vi "配置写入.vi"(8 "error in (no error)":errorcluster caption="错误输入（无错误）") -> (0 "错误输出":errorcluster)   [LabVIEW 2022 SP3, in "斯坦道氨氮V2.lvlib"]
uses:
  <vilib>/Utility/config.llb/NI_LVConfig.lvlib
  <userlib>/_OpenG.lib/variantconfig/variantconfig.llb/openg_variant_configuration_file.lvlib
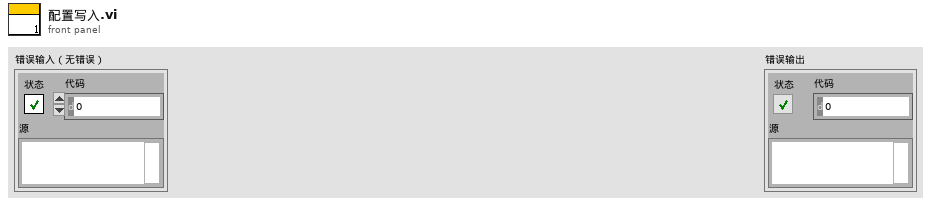
[diagram p1: front panel]
types:
  T1 = typedef "NI_LVConfig.lvlib/Config Data RefNum.ctl" = refnum<k1>
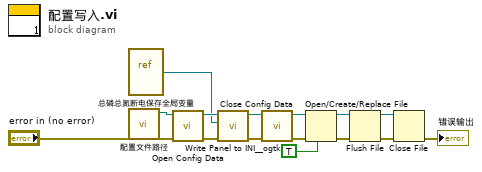
[diagram p0: block diagram]
diagram:
  n1 = vi-ref "总磷总氮断电保存全局变量.vi"() -> (w14:refnum<vi>)
  n2 = call "配置文件路径.vi"() -> ("appended path"=w2:path)  [unwired: 11 in]
  n3 = call <vilib>:"Open Config Data.vi"("error in (no error)"="error in (no error)", "configuration file path"=w2) -> ("error out"=w12:errorcluster, "refnum"=w15:T1)  [unwired: 7 in, 1 out]
  n4 = call <userlib>:"Write Panel to INI__ogtk.vi"("error in (no error)"=w12, "VI ref"=w14, "refnum"=w15) -> ("error out"=w11:errorcluster, "refnum out"=w13:T1)  [unwired: 7 in]
  n5 = call <vilib>:"Close Config Data.vi"("error in (no error)"=w11, "refnum"=w13) -> ("error out"=w6:errorcluster, "file path"=w5:path)  [unwired: 8 in]
  n6 = Open/Create/Replace File(file path (use dialog)=w5, error in=w6, disable buffering (F)=TRUE ("禁用缓存(F)")) -> (refnum out=w9:refnum<file>, error out=w10:errorcluster)  [unwired: 3 in, 1 out]
  n7 = Flush File(refnum=w9, error in=w10) -> (refnum out=w8:refnum<file>, error out=w7:errorcluster)
  n8 = Close File(refnum=w8, error in=w7) -> (error out=→"错误输出":errorcluster)  [unwired: 1 out]
